vi "Force Sensors.vi"() -> ()   [LabVIEW 2018]
uses:
  <vilib>/Instr/_visa.llb/VISA Configure Serial Port (Instr).vi
  <vilib>/ptbypt/NI_PtbyPt.lvlib
panel:
  out "Force in Newtons":dbl(graph)
  out "Force in Newtons":dbl(graph)
  in  "COM Port-Sensor 2":refnum<visa-resource-name>="COM1"
  out "Sensor Raw Value 2":i32
  out "Force in Kilograms":dbl(graph)
  out "Force in Kilograms":dbl(graph)
  out "Sensor Raw Value":i32
  in  "COM Port-Sensor 1":refnum<visa-resource-name>="COM1"
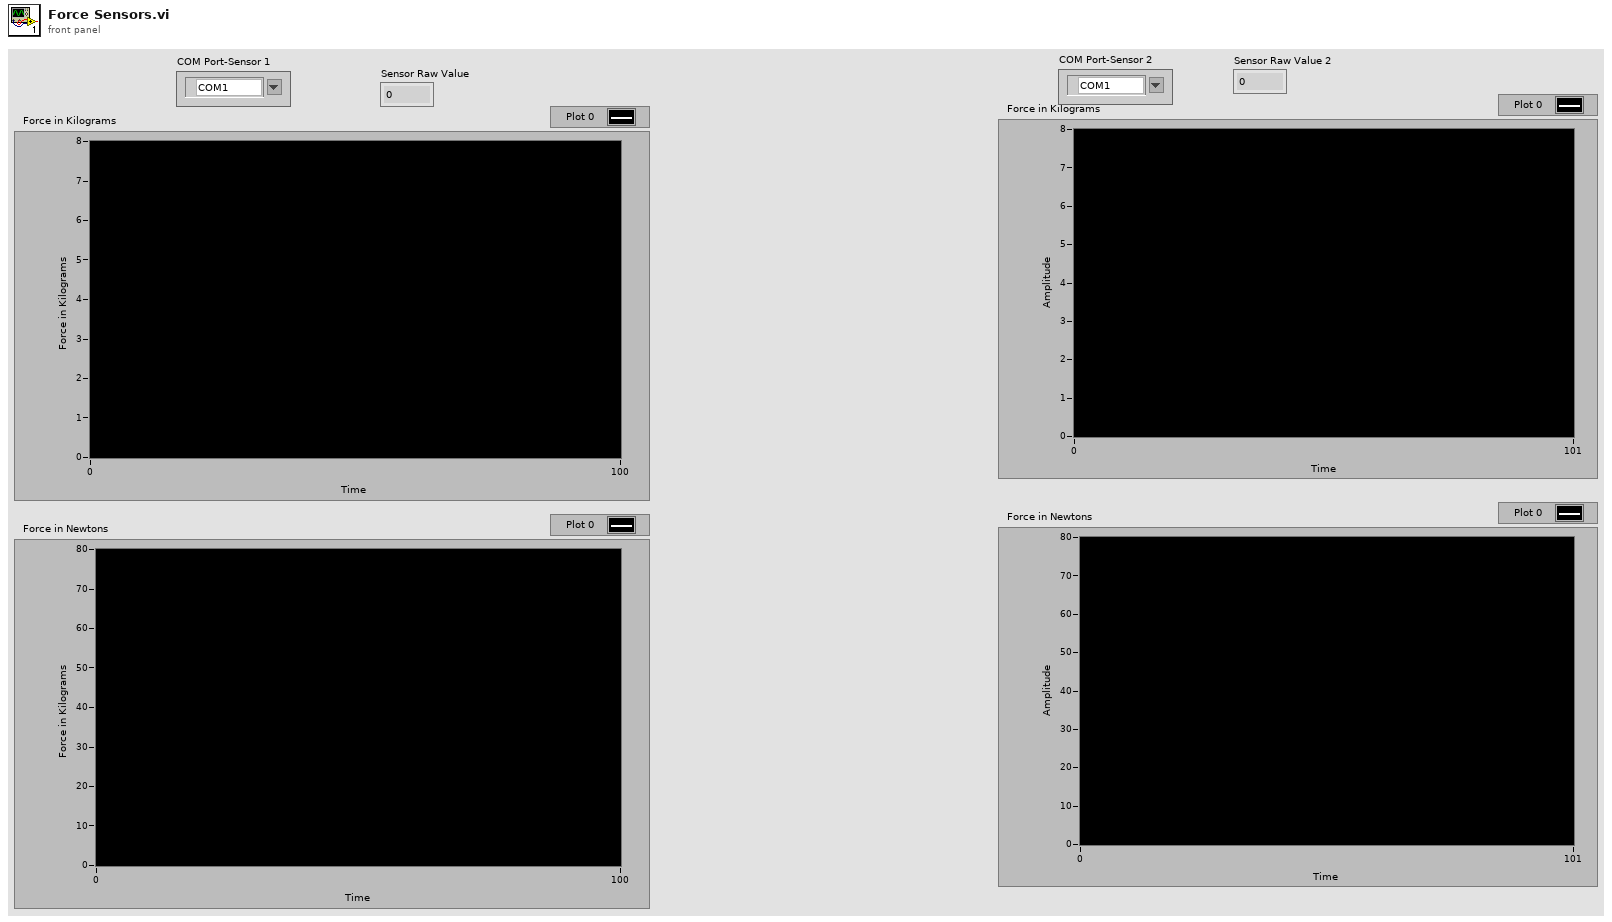
[diagram p1: front panel]
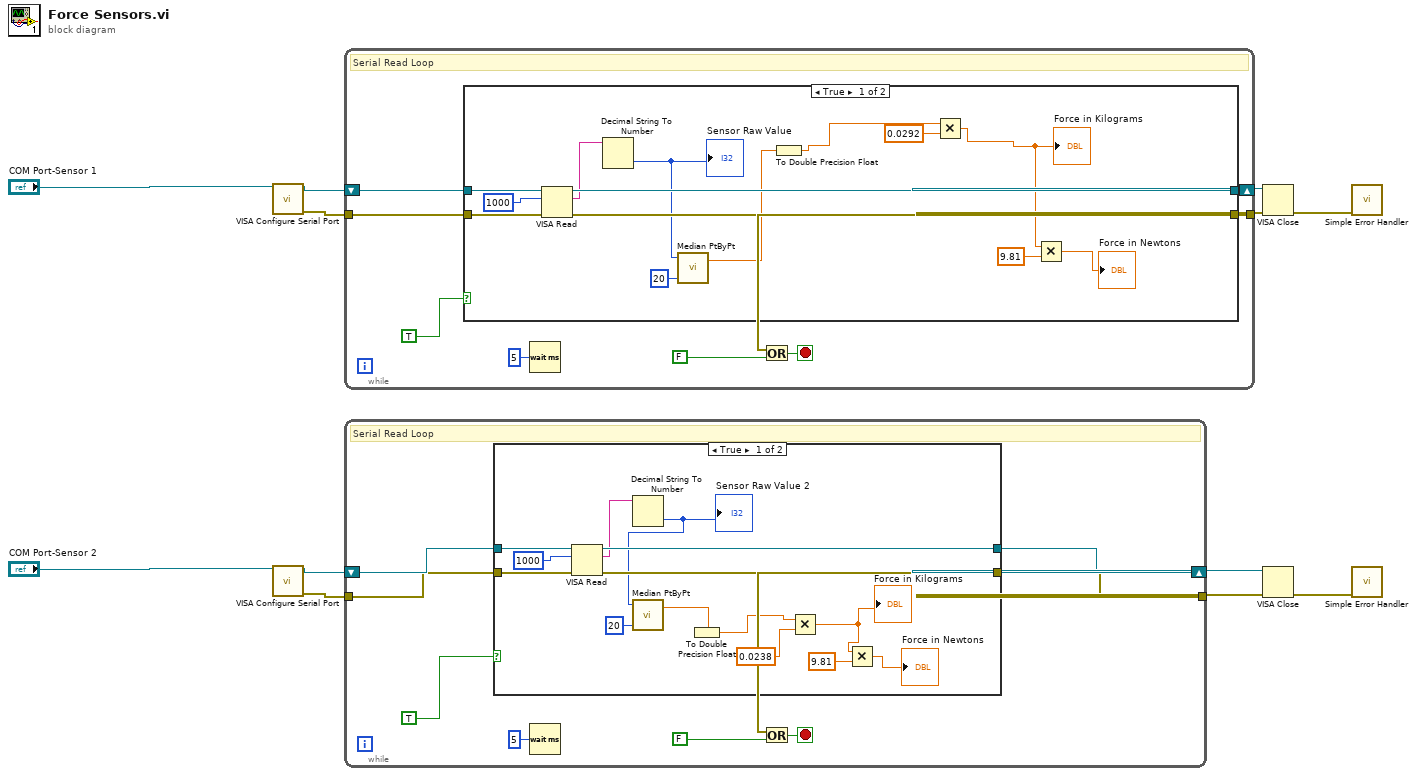
[diagram p0: block diagram]
diagram:
  n1 = call-poly "VISA Configure Serial Port"("VISA resource name"="COM Port-Sensor 1") -> ("VISA resource name out"=w8:refnum<visa-resource-name>, "error out"=w7:errorcluster)  [unwired: 9 in, 4 out]
  n2 = call-poly "VISA Configure Serial Port"("VISA resource name"="COM Port-Sensor 2") -> ("VISA resource name out"=w2:refnum<visa-resource-name>, "error out"=w1:errorcluster)  [unwired: 9 in, 4 out]
  n3 = while {
    shift-right: [w20] -> w9
    shift-left: w8 -> [w16]
    tunnel: w7 -> [w15]
    tunnel: [w17] -> w10
    stop <- w18 stop-if-true
    # "Serial Read Loop"
    n4 = case shown="True" TRUE {
      tunnel: [w32 w36] -> w20
      tunnel: w16 -> [w34 w36]
      tunnel: [w31 w35] -> w17
      tunnel: w15 -> [w33 w35]
      frame True {
        n5 = VISA Read(VISA resource name=w34, byte count=u32 1000, error in (no error)=w33) -> (VISA resource name out=w32:refnum<visa-resource-name>, read buffer=w29:string, error out=w31:errorcluster)  [unwired: 1 out]
        n6 = Decimal String To Number(string=w29) -> (number=w27:i32)  [unwired: 2 in, 1 out]
        "Sensor Raw Value" <- w27
        n7 = call <vilib>:"Median PtByPt.vi"("sample length"=20, "x"=w27) -> ("median"=w25:dbl)  [unwired: 2 in, 1 out]
        n8 = To Double Precision Float(number=w25) -> (double precision float=w21:dbl)
        n9 = Multiply(x=w21, y=0.0292) -> (x*y=w24:dbl)
        "Force in Kilograms" <- w24
        n10 = Multiply(x=w24, y=9.81) -> (x*y=→"Force in Newtons":dbl)
      }
      frame False {
      }
    }
    n11 = Wait (ms)(milliseconds to wait=u32 5) -> ()  [unwired: 1 out]
    n12 = Or(x=w17, y=FALSE) -> (x .or. y?=w18:bool)
  }
  n13 = while {
    shift-right: [w44] -> w3
    shift-left: w2 -> [w40]
    tunnel: w1 -> [w39]
    tunnel: [w41] -> w4
    stop <- w42 stop-if-true
    # "Serial Read Loop"
    n14 = case shown="True" TRUE {
      tunnel: [w56 w60] -> w44
      tunnel: w40 -> [w58 w60]
      tunnel: [w55 w59] -> w41
      tunnel: w39 -> [w57 w59]
      frame True {
        n15 = VISA Read(VISA resource name=w58, byte count=u32 1000, error in (no error)=w57) -> (VISA resource name out=w56:refnum<visa-resource-name>, read buffer=w53:string, error out=w55:errorcluster)  [unwired: 1 out]
        n16 = Decimal String To Number(string=w53) -> (number=w49:i32)  [unwired: 2 in, 1 out]
        "Sensor Raw Value 2" <- w49
        n17 = call <vilib>:"Median PtByPt.vi"("sample length"=20, "x"=w49) -> ("median"=w50:dbl)  [unwired: 2 in, 1 out]
        n18 = To Double Precision Float(number=w50) -> (double precision float=w46:dbl)
        n19 = Multiply(x=w46, y=0.0238) -> (x*y=w45:dbl)
        "Force in Kilograms" <- w45
        n20 = Multiply(x=w45, y=9.81) -> (x*y=→"Force in Newtons":dbl)
      }
      frame False {
      }
    }
    n21 = Wait (ms)(milliseconds to wait=u32 5) -> ()  [unwired: 1 out]
    n22 = Or(x=w41, y=FALSE) -> (x .or. y?=w42:bool)
  }
  n23 = VISA Close(VISA resource name=w9, error in (no error)=w10) -> (error out=w11:errorcluster)
  n24 = VISA Close(VISA resource name=w3, error in (no error)=w4) -> (error out=w5:errorcluster)
  n25 = call <vilib>:"Simple Error Handler.vi"("error in (no error)"=w11) -> ()  [unwired: 1 in, 8 out]
  n26 = call <vilib>:"Simple Error Handler.vi"("error in (no error)"=w5) -> ()  [unwired: 1 in, 8 out]
